vi "Main UI.vi"(8 "error in (no error)":errorcluster, 11 "App in":refnum<class "App.lvclass">) -> (0 "error out":errorcluster, 3 "App out":refnum<class "App.lvclass">)   [LabVIEW 2020, in "PicoG-App.lvlib" / "App.lvclass"]
uses:
  App.lvclass
  UI State.ctl
  App.lvclass/App.ctl
  Main UI Events.ctl
  Popout Nav Panel Event.ctl
  <vilib>/IlluminatedG/IG OOPanel/OOPanel/Panel/Panel.lvclass
  App Watcher/App Update Data.ctl
  ViaApp/ViaApp.lvclass
  AppListPanel/AppListPanel.lvclass
  C:/Program Files (x86)/National Instruments/LabVIEW 2020/vi.lib/IlluminatedG/IG OOPanel/OOPanel/Panel/Panel.lvclass
  C:/dev/Vireo/PicoG/PicoG-App/NavPanel/NavPanel.lvclass
  DeviceListPanel/DeviceListPanel.lvclass
  PlatformListPanel/PlatformListPanel.lvclass
  NavPanel/NavPanel.lvclass
  <vilib>/Utility/cursorutil.llb/Set Cursor (Icon Pict).vi
  <vilib>/IlluminatedG/IG OOPanel/OOPanel/Manager/Manager.lvclass
  PicoG-App.lvlib
  App Watcher/App Watcher.lvclass
panel:
  in  "Devices":bool
  in  "Apps":bool
  in  "Platforms":bool
  out "StatusLeft":string
  out "StatusLeft 2":string
  out "StatusRight 2":string
  out "ProgressBar":dbl(slide) scale=0.0..100.0
  out "StatusRight":string
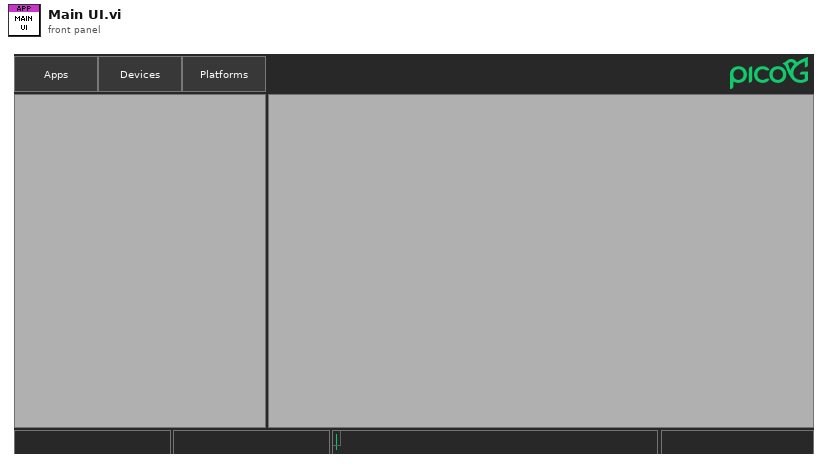
[diagram p1: front panel]
types:
  T1 = typedef "PicoG-App.lvlib/App.lvclass/UI State.ctl" = enum16{"Init", "Run", "Close"}
  T2 = enum32{"Invalid", "Standard", "Closed", "Hidden", "Minimized", "Maximized"}
  T3 = typedef "PicoG-App.lvlib/App.lvclass/Main UI Events.ctl" = cluster{"Popout Nav Event":refnum<user-event>, "Add App":refnum<user-event>, "App Update":refnum<user-event>}
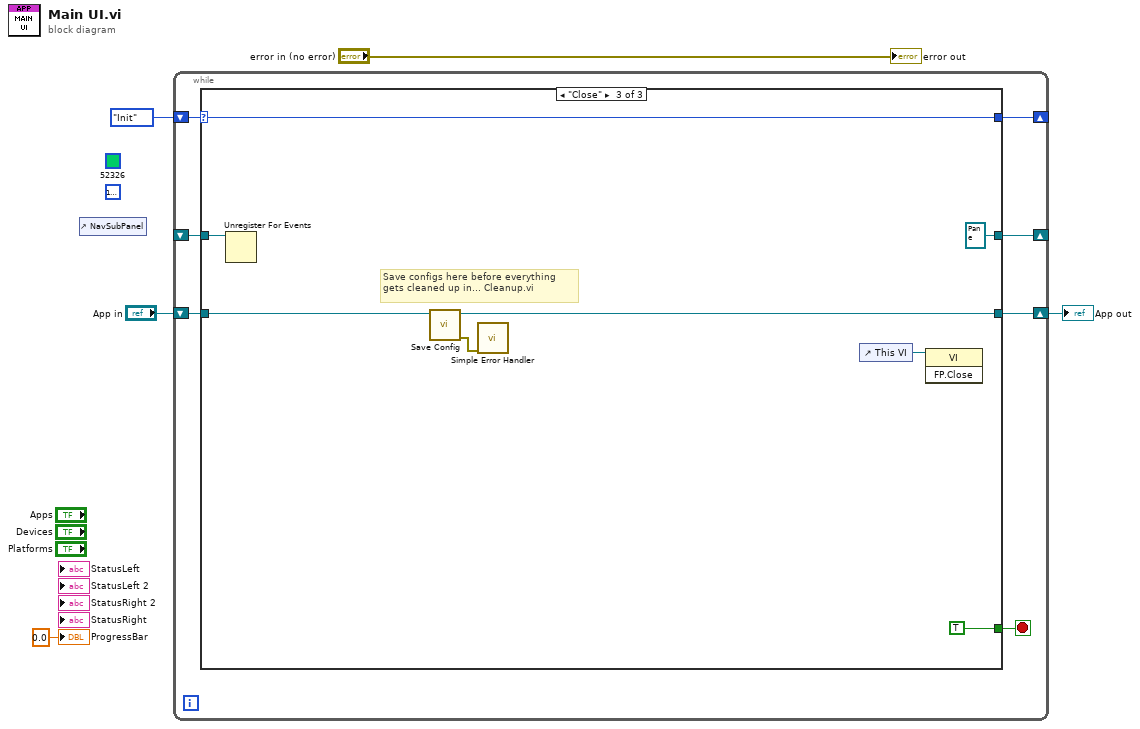
[diagram p0: block diagram]
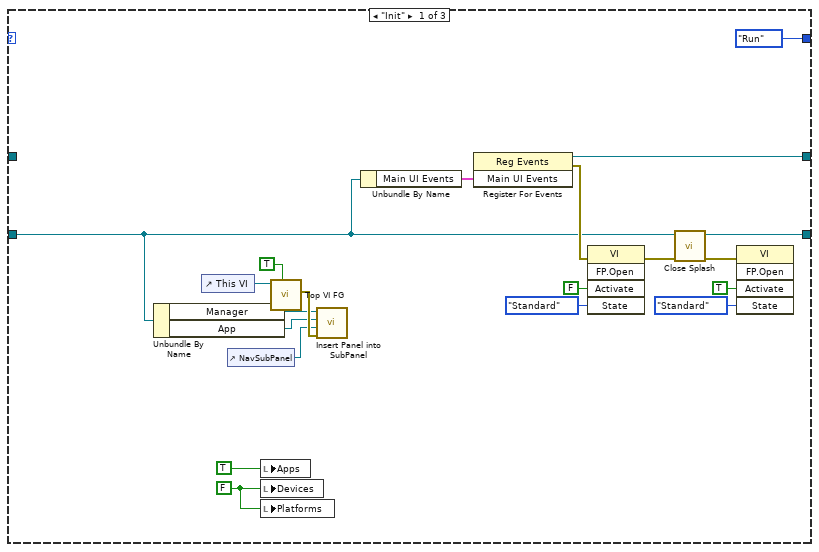
[diagram p2: hidden frame]
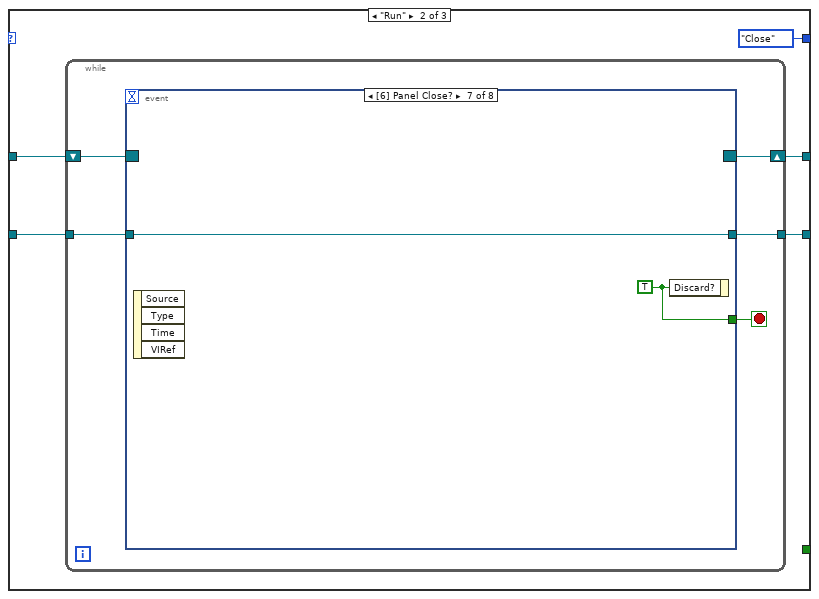
[diagram p3: hidden frame]
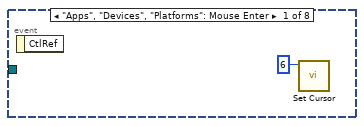
[diagram p4: hidden frame]
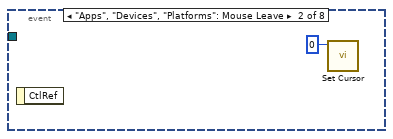
[diagram p5: hidden frame]
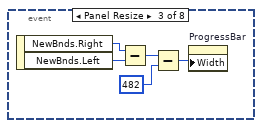
[diagram p6: hidden frame]
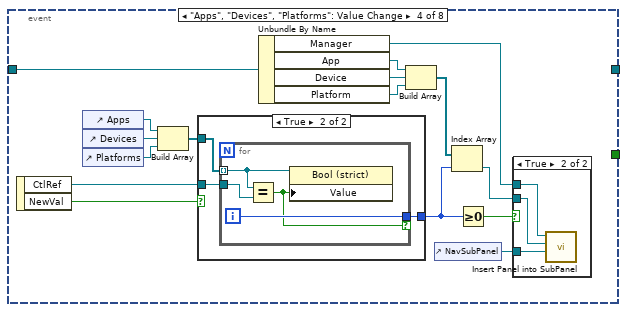
[diagram p7: hidden frame]
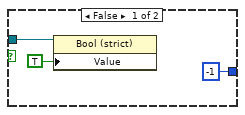
[diagram p9: hidden frame]
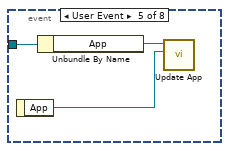
[diagram p10: hidden frame]
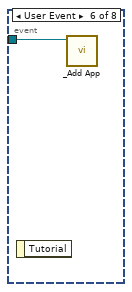
[diagram p11: hidden frame]
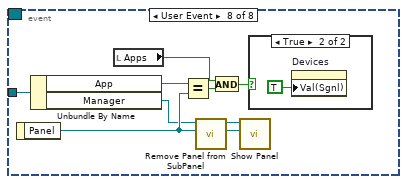
[diagram p12: hidden frame]
diagram:
  (unwired) u32 16777216
  (unwired) u32 52326
  n1 = control-ref of="NavSubPanel"() -> ()  [unwired: 1 out]
  n2 = while {
    shift-right: [w11] -> _
    shift-left: UI_State."Init" ("UI State") -> [w12]
    shift-right: [w8] -> w2
    shift-left: "App in" -> [w9]
    shift-right: [w7] -> _
    shift-left: _ -> [w6]
    stop <- w10 stop-if-true
    n3 = case shown="\"Close\"" w12 {
      selector: w12 -> [_ _ w102]
      tunnel: [UI_State."Run" ("UI State") UI_State."Close" ("UI State") w102] -> w11
      tunnel: [_ _ TRUE] -> w10
      tunnel: w9 -> [w17 w36 w97]
      tunnel: [w23 w35 w96] -> w8
      tunnel: [w20 w33 refnum<event-registration> refnum ("Event Registration Refnum")] -> w7
      tunnel: w6 -> [_ w34 w99]
      frame "Init" {
        w13 = FALSE ("Nav Devices")
        n4 = Unbundle By Name(w17) -> ("Manager"=w16:refnum<class "Manager.lvclass">, "App"=w15:refnum<class "AppListPanel.lvclass">)
        n5 = control-ref of="This VI"() -> (w19:refnum<vi>)
        n6 = control-ref of="NavSubPanel"() -> (w22:refnum<vi>)
        n7 = local write "Apps"(TRUE ("Nav Apps")) -> ()
        n8 = local write "Devices"(w13) -> ()
        n9 = local write "Platforms"(w13) -> ()
        n10 = call "Top VI FG.vi"("Set (F)"=TRUE, "Top-Level VI In"=w19) -> ("error out"=w32:errorcluster)  [unwired: 8 in, 1 out]
        n11 = call <vilib>:"Insert Panel into SubPanel.vi"("error in (no error)"=w32, "SubPanel"=w22, "Panel In"=w15, "Manager in"=w16) -> ()  [unwired: 5 in, 3 out]
        n12 = Unbundle By Name(w17) -> ("Main UI Events"=w21:T3)
        n13 = register-events(w21) -> (reference out=w20:refnum<event-registration>, error out=w31:errorcluster)  [unwired: 2 in]
        n14 = invoke class="VI" method="FP.Open"(error in=w31, "Activate"=FALSE ("Activate?"), "State"=T2."Standard") -> (error out=w27:errorcluster)  [unwired: 2 in, 4 out]
        n15 = call "Close Splash.vi"("error in (no error)"=w27, "App in"=w17) -> ("error out"=w26:errorcluster, "App out"=w23:refnum<class "App.lvclass">)  [unwired: 8 in]
        n16 = invoke class="VI" method="FP.Open"(error in=w26, "Activate"=TRUE ("Activate?"), "State"=T2."Standard") -> ()  [unwired: 2 in, 5 out]
      }
      frame "Run" {
        n17 = while {
          tunnel: w36 -> [w41]
          tunnel: [w40] -> w35
          shift-right: [w38] -> w33
          shift-left: w34 -> [w39]
          stop <- w42 stop-if-true
          n18 = event shown="[6] Panel Close?" {
            selector: w39 -> [_ _ _ _ _ _ _ _]
            dyn-events: [_ _ _ _ _ _ _ _] -> w38
            timeout: _ -> [_ _ _ _ _ _ _ _]
            tunnel: [_ _ _ _ _ _ w84 _] -> w42
            tunnel: w41 -> [_ _ _ w56 w81 w82 w83 w87]
            tunnel: [_ _ _ _ _ _ w83 _] -> w40
            event "Apps", "Devices", "Platforms": Mouse Enter {
              n19 = event-data() -> ()  [unwired: 1 in, 1 out]
              n20 = call-poly <vilib>:"Set Cursor.vi"("icon"=u16 6) -> ()  [unwired: 9 in, 2 out]
            }
            event "Apps", "Devices", "Platforms": Mouse Leave {
              n21 = event-data() -> ()  [unwired: 1 in, 1 out]
              n22 = call-poly <vilib>:"Set Cursor.vi"("icon"=u16 0) -> ()  [unwired: 9 in, 2 out]
            }
            event Panel Resize {
              n23 = event-data() -> ("NewBnds.Right"=w48:i16, "NewBnds.Left"=w49:i16)  [unwired: 1 in]
              n24 = Subtract(x=w48, y=w49) -> (x-y=w47:i16)
              n25 = Subtract(x=w47, y=i16 482) -> (x-y=w45:i16)
              n26 = property on="ProgressBar" class="Slide (strict)"("Width"=w45) -> ()  [unwired: 2 in, 2 out]
            }
            event "Apps", "Devices", "Platforms": Value Change {
              n27 = event-data() -> ("CtlRef"=w64:refnum<vi>, "NewVal"=w65:bool)  [unwired: 1 in]
              n28 = control-ref of="Apps"() -> (w62:refnum<vi>)
              n29 = control-ref of="Devices"() -> (w63:refnum<vi>)
              n30 = control-ref of="Platforms"() -> (w61:refnum<vi>)
              n31 = Build Array(w62, w63, w61) -> (w50:refnum<vi>[])
              n32 = case shown="True" w65 {
                tunnel: w64 -> [w71 w74]
                tunnel: w50 -> [_ w73]
                tunnel: [-1 w72] -> w60
                frame False {
                  n33 = property class="Bool (strict)"(reference=w71, "Value"=TRUE) -> ()  [unwired: 1 in, 2 out]
                }
                frame True {
                  n34 = for {
                    tunnel: w74 -> [w78]
                    tunnel: w73 -> [w77] mode=indexing
                    tunnel: [w76] -> w72 if=w75
                    i -> [w76]
                    n35 = Equal?(x=w77, y=w78) -> (x = y?=w75:bool)
                    n36 = property class="Bool (strict)"(reference=w77, "Value"=w75) -> ()  [unwired: 1 in, 2 out]
                  }
                }
              }
              n37 = Unbundle By Name(w56) -> ("Manager"=w51:refnum<class "Manager.lvclass">, "App"=w54:refnum<class "AppListPanel.lvclass">, "Device"=w55:refnum<class "DeviceListPanel.lvclass">, "Platform"=w53:refnum<class "PlatformListPanel.lvclass">)
              n38 = Build Array(w54, w55, w53) -> (w52:refnum<class "NavPanel.lvclass">[])
              n39 = control-ref of="NavSubPanel"() -> (w58:refnum<vi>)
              n40 = Index Array(array=w52, index=w60) -> (element=w57:refnum<class "NavPanel.lvclass">)
              n41 = Greater Or Equal To 0?(x=w60) -> (x >= 0?=w59:bool)
              n42 = case shown="True" w59 {
                tunnel: w58 -> [_ w68]
                tunnel: w57 -> [_ w67]
                tunnel: w51 -> [_ w66]
                frame False {
                }
                frame True {
                  n43 = call <vilib>:"Insert Panel into SubPanel.vi"("SubPanel"=w68, "Panel In"=w67, "Manager in"=w66) -> ()  [unwired: 6 in, 3 out]
                }
              }
            }
            event User Event {
              n44 = event-data() -> ("App"=w79:refnum<class "ViaApp.lvclass">)  [unwired: 1 in]
              n45 = Unbundle By Name(w81) -> ("App"=w80:refnum<class "AppListPanel.lvclass">)
              n46 = call "Update App.vi"("ViaApp"=w79, "AppListPanel in"=w80) -> ()  [unwired: 8 in, 2 out]
            }
            event User Event {
              n47 = event-data() -> ()  [unwired: 1 in, 1 out]
              n48 = call "_Add App.vi"("App in"=w82) -> ()  [unwired: 9 in, 2 out]
            }
            event Panel Close? {
              w84 = TRUE ("Discard?")
              n49 = event-data() -> ()  [unwired: 1 in, 4 out]
              n50 = event-data("Discard?"=w84) -> ()  [unwired: 1 in, 1 out]
            }
            event User Event {
              n51 = event-data() -> ("Panel"=w89:refnum<class "Panel.lvclass">)  [unwired: 1 in]
              n52 = Unbundle By Name(w87) -> ("App"=w86:refnum<class "AppListPanel.lvclass">, "Manager"=w85:refnum<class "Manager.lvclass">)
              n53 = local read "Apps"() -> (w90:bool)
              n54 = Equal?(x=w86, y=w89) -> (x = y?=w91:bool)
              n55 = call <vilib>:"Remove Panel from SubPanel.vi"("Panel In"=w89, "Manager in"=w85) -> ("Panel"=w92:refnum<class "Panel.lvclass">, "Manager out"=w93:refnum<class "Manager.lvclass">)  [unwired: 7 in, 1 out]
              n56 = And(x=w90, y=w91) -> (x .and. y?=w88:bool)
              n57 = call <vilib>:"Show Panel.vi"("Panel In"=w92, "Manager in"=w93) -> ()  [unwired: 7 in, 3 out]
              n58 = case shown="True" w88 {
                frame False {
                }
                frame True {
                  n59 = property on="Devices" class="Bool (strict)"("Val(Sgnl)"=TRUE ("Value (Signaling)")) -> ()  [unwired: 2 in, 2 out]
                }
              }
            }
          }
        }
      }
      frame "Close" {
        # "Save configs here before everything gets cleaned up in... Cleanup.vi"
        n60 = Unregister For Events(event registration refnum=w99) -> ()  [unwired: 1 in, 1 out]
        n61 = call "Save Config.vi"("App in"=w97) -> ("error out"=w95:errorcluster, "App out"=w96:refnum<class "App.lvclass">)  [unwired: 9 in]
        n62 = call <vilib>:"Simple Error Handler.vi"("error in (no error)"=w95) -> ()  [unwired: 4 in, 5 out]
        n63 = control-ref of="This VI"() -> (w100:refnum<vi>)
        n64 = invoke class="VI" method="FP.Close"(reference=w100) -> ()  [unwired: 2 in, 3 out]
      }
    }
  }
  "App out" <- w2
  "error out" <- "error in (no error)"
  "ProgressBar" <- 0.0 ("ProgressBar")
